vi "LecturaBluefors.vi"() -> ()   [LabVIEW 2017]
uses:
  Temperaturas Bluefors.ctl
panel:
  out "Canal":i32
  out "Numeric":i32
  out "datoNuevo?":bool=TRUE
  in  "Web(T)":bool=TRUE
  out "date/time string":string
  out "error out":errorcluster
  in  "error in (no error)":errorcluster
  in  "url":string="http://192.168.0.101:5001/channel/measurement/latest"
  in  "stop":bool
  in  "Delay":dbl
  out "BLUEFORS":T1 {"Canal 8" format="%.3f"; "Canal 7" format="%.3f"; "Canal 6" format="%.3f"; "Canal 5" format="%.3f"; "Canal 4" format="%.3f"; "Canal 3" format="%.3f"; "Canal 2" format="%.3f"; "Canal 1" format="%.3f"}
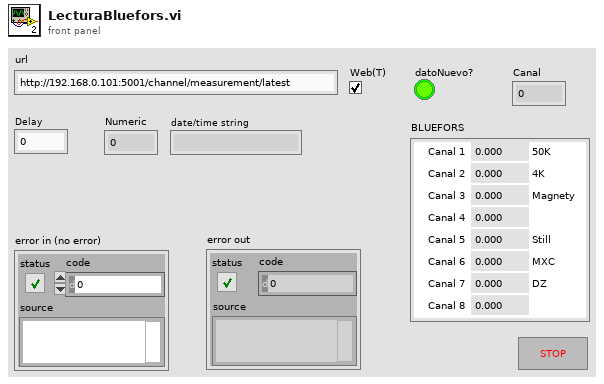
[diagram p1: front panel]
types:
  T1 = typedef "Temperaturas Bluefors.ctl" = cluster{"Canal 1":dbl, "Canal 2":dbl, "Canal 3":dbl, "Canal 4":dbl, "Canal 5":dbl, "Canal 6":dbl, "Canal 7":dbl, "Canal 8":dbl}
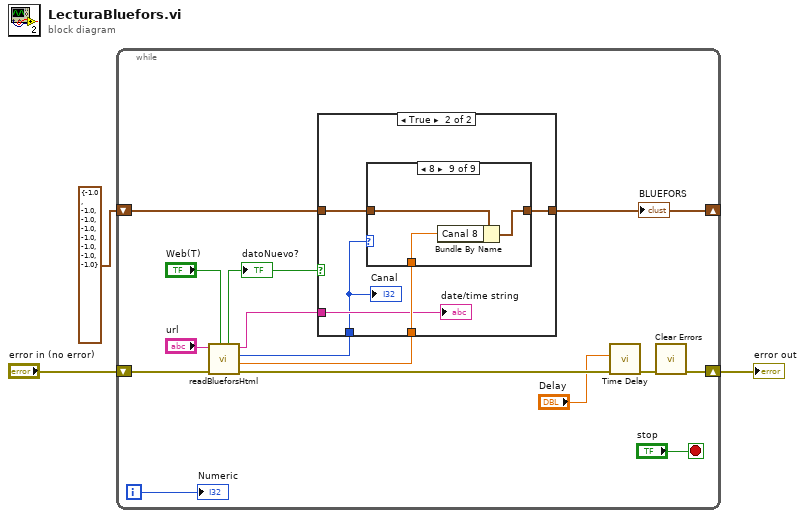
[diagram p0: block diagram]
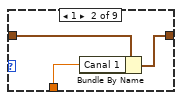
[diagram p4: hidden frame]
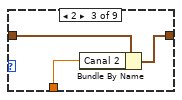
[diagram p5: hidden frame]
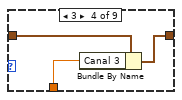
[diagram p6: hidden frame]
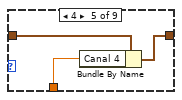
[diagram p7: hidden frame]
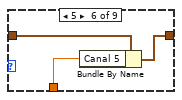
[diagram p8: hidden frame]
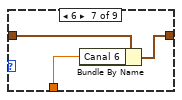
[diagram p9: hidden frame]
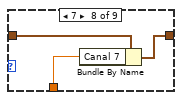
[diagram p10: hidden frame]
diagram:
  n1 = while {
    shift-right: [w16] -> _
    shift-left: T1 {"Canal 1"=-1.0, "Canal 2"=-1.0, "Canal 3"=-1.0, "Canal 4"=-1.0, "Canal 5"=-1.0, "Canal 6"=-1.0, "Canal 7"=-1.0, "Canal 8"=-1.0} ("BLUEFORS") -> [w17]
    shift-right: [w13] -> w2
    shift-left: "error in (no error)" -> [w15]
    i -> [w7]
    stop <- "stop" stop-if-true
    n2 = call "readBlueforsHtml.vi"("Web(T)"="Web(T)", "Error In"=w15, "url"="url") -> ("Error Out"=w14:errorcluster, "temperatura"=w10:dbl, "chan_nr"=w11:i32, "date/time string"=w4:string, "datoNuevo?"=w8:bool)  [unwired: 3 in, 1 out]
    "datoNuevo?" <- w8
    n3 = case shown="True" w8 {
      tunnel: w17 -> [w19 w24]
      tunnel: [w19 w23] -> w16
      tunnel: w11 -> [_ w20]
      tunnel: w10 -> [_ w22]
      tunnel: w4 -> [_ w21]
      frame False {
      }
      frame True {
        n4 = case shown="8" w20 {
          tunnel: w24 -> [w25 w28 w31 w34 w37 w40 w43 w46 w49]
          tunnel: [w25 w27 w30 w33 w36 w39 w42 w45 w48] -> w23
          tunnel: w22 -> [_ w26 w29 w32 w35 w38 w41 w44 w47]
          frame 0, Default {
          }
          frame 1 {
            n5 = Bundle By Name(cluster=w28, "Canal 1"=w26) -> (w27:T1)
          }
          frame 2 {
            n6 = Bundle By Name(cluster=w31, "Canal 2"=w29) -> (w30:T1)
          }
          frame 3 {
            n7 = Bundle By Name(cluster=w34, "Canal 3"=w32) -> (w33:T1)
          }
          frame 4 {
            n8 = Bundle By Name(cluster=w37, "Canal 4"=w35) -> (w36:T1)
          }
          frame 5 {
            n9 = Bundle By Name(cluster=w40, "Canal 5"=w38) -> (w39:T1)
          }
          frame 6 {
            n10 = Bundle By Name(cluster=w43, "Canal 6"=w41) -> (w42:T1)
          }
          frame 7 {
            n11 = Bundle By Name(cluster=w46, "Canal 7"=w44) -> (w45:T1)
          }
          frame 8 {
            n12 = Bundle By Name(cluster=w49, "Canal 8"=w47) -> (w48:T1)
          }
        }
        "date/time string" <- w21
        "Canal" <- w20
      }
    }
    "BLUEFORS" <- w16
    n13 = call "Time Delay"("error in (no error)"=w14, "Delay Time (s)"="Delay") -> ("error out"=w6:errorcluster)  [unwired: 9 in]
    n14 = call <vilib>:"Clear Errors.vi"("error in (no error)"=w6) -> ("error out"=w13:errorcluster)  [unwired: 5 in, 1 out]
    "Numeric" <- w7
  }
  "error out" <- w2
